vi "stoperaseDO_img.vi"   [LabVIEW 2015]
uses:
  waveforms/usedDOindepofwf.vi
  Objects/2pparameters.vi
  Objects/configuration.vi
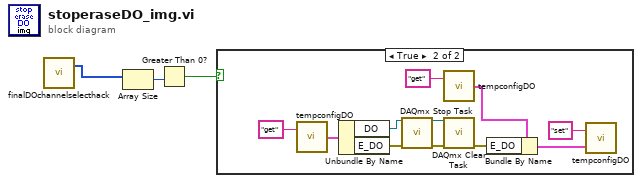
[diagram p0: block diagram]
diagram:
  n1 = call "finalDOchannelselecthack.vi"() -> ("usedDO"=w1:u32[])  [unwired: 1 in, 1 out]
  n2 = Array Size(array=w1) -> (size(s)=w3:i32)
  n3 = Greater Than 0?(x=w3) -> (x > 0?=w2:bool)
  n4 = case shown="True" w2 {
    frame False {
    }
    frame True {
      n5 = call "tempconfigDO.vi"("command"="get") -> ("Temp Config out"=w11:cluster{"DO":refnum<k21>, "E_DO":errorcluster})  [unwired: 1 in]
      n6 = Unbundle By Name(w11) -> ("DO"=w10:refnum<k21>, "E_DO"=w9:errorcluster)
      n7 = call <vilib>:"DAQmx Stop Task.vi"("task/channels in"=w10, "error in"=w9) -> ("task out"=w6:refnum<k21>, "error out"=w5:errorcluster)  [unwired: 12 in]
      n8 = call "tempconfigDO.vi"("command"="get") -> ("Temp Config out"=w8:cluster{"DO":refnum<k21>, "E_DO":errorcluster})  [unwired: 1 in]
      n9 = call <vilib>:"DAQmx Clear Task.vi"("task in"=w6, "error in"=w5) -> ("error out"=w4:errorcluster)  [unwired: 13 in]
      n10 = Bundle By Name(cluster=w8, "E_DO"=w4) -> (w7:cluster{"DO":refnum<k21>, "E_DO":errorcluster})
      n11 = call "tempconfigDO.vi"("Temp Config in"=w7, "command"="set") -> ()  [unwired: 1 out]
    }
  }
